vi "P2PSendData.vi"(8 "error in (no error)":errorcluster, 9 "DataExchange":T1, 10 "TargetDeviceEnqueuer":refnum<class "Message Enqueuer.lvclass">, 11 "DataGenerator in":refnum<class "DataGenerator.lvclass">) -> (0 "error out":errorcluster, 3 "DataGenerator out":refnum<class "DataGenerator.lvclass">)   [LabVIEW 2020, in "DataGenerator.lvclass"]
uses:
  DataGenerator.lvclass
  Model/Hardware Abstraction Layer/Component/Device/Device/DataExchange.ctl
  <vilib>/ActorFramework/Message Enqueuer/Message Enqueuer.lvclass
  DataListener/DataListener.lvclass
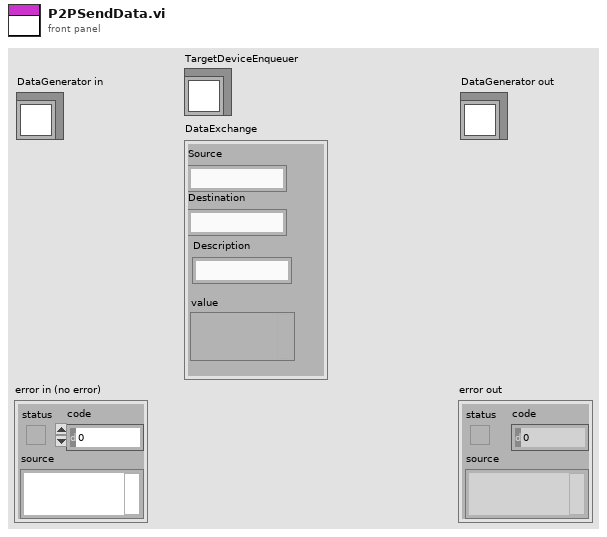
[diagram p1: front panel]
types:
  T1 = typedef "DataListener.lvclass/DataExchange.ctl" = cluster{"Source":string, "Destination":string, "Description":string, "value":variant}
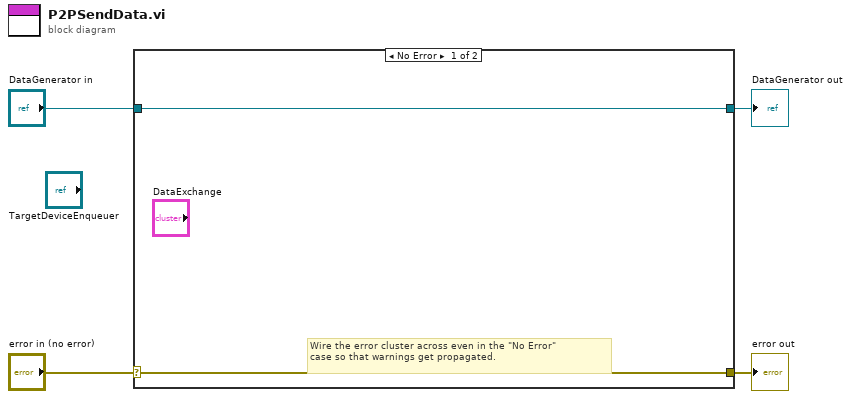
[diagram p0: block diagram]
diagram:
  n1 = case shown="No Error" "error in (no error)" {
    selector: "error in (no error)" -> [w5 w8]
    tunnel: [w5 w8] -> w3
    tunnel: [w6 w7] -> w1
    tunnel: "DataGenerator in" -> [w6 w7]
    frame No Error {
      # "Wire the error cluster across even in the \"No Error\"\ncase so that warnings get propagated."
    }
    frame Error {
    }
  }
  "error out" <- w3
  "DataGenerator out" <- w1
